vi "CollectData.vi"(8 "error in (no error)":errorcluster, 11 "SRS_DS345 in":refnum<class "SRS_DS345.lvclass">) -> (0 "error out":errorcluster, 3 "SRS_DS345 out":refnum<class "SRS_DS345.lvclass">)   [LabVIEW 2013, in "SRS_DS345.lvclass"]
uses:
  SRS_DS345.lvclass
  Device/Device.lvclass
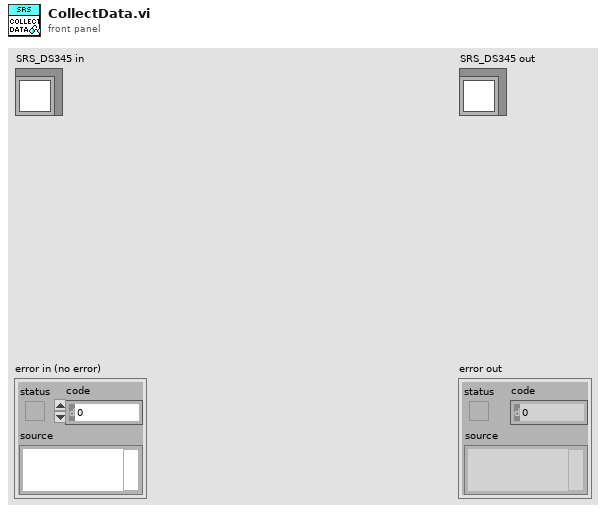
[diagram p1: front panel]
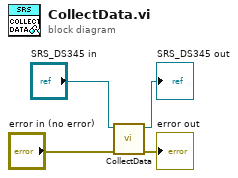
[diagram p0: block diagram]
diagram:
  n1 = call-parent "CollectData.vi"("error in (no error)"="error in (no error)", "Device in"="SRS_DS345 in") -> ("error out"=→"error out":errorcluster, "Device out"=→"SRS_DS345 out":refnum<class "SRS_DS345.lvclass">)  [unwired: 8 in]
